vi "Timer enkoder update.vi"(7 "Akcja (Get T)":T1=enum."Get Time", 8 "error in (no error)":errorcluster, 10 "Set Time":dbl) -> (0 "error out":errorcluster, 2 "Get Time":dbl, 3 "Elapsed?":bool)   [LabVIEW 2014]
doc: "Use this template to build a VI to use as a subVI."
uses:
  Kontrolki/FVGs/FGV Timer akcje.ctl
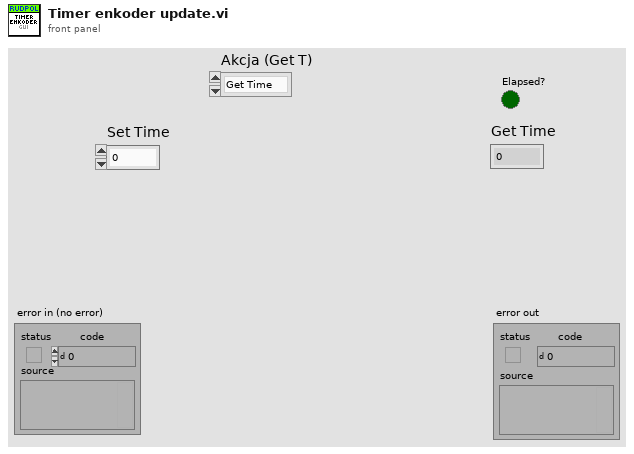
[diagram p1: front panel]
types:
  T1 = typedef "FGV Timer akcje.ctl" = enum16{"Reset", "Get Time"}
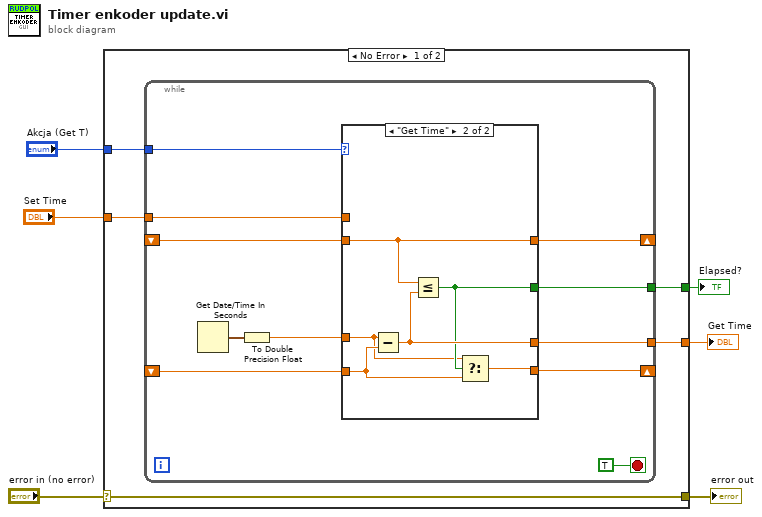
[diagram p0: block diagram]
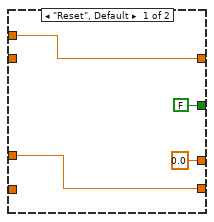
[diagram p2: hidden frame]
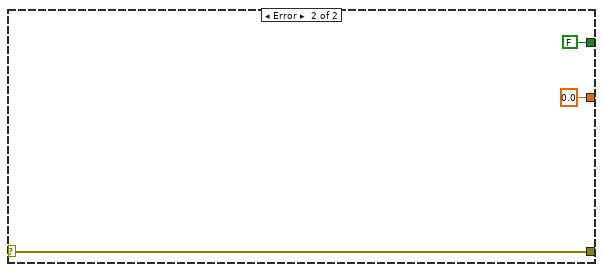
[diagram p3: hidden frame]
diagram:
  n1 = case shown="No Error" "error in (no error)" {
    selector: "error in (no error)" -> [w11 w35]
    tunnel: [w11 w35] -> w5
    tunnel: "Akcja (Get T)" -> [w10 _]
    tunnel: "Set Time" -> [w9 _]
    tunnel: [w8 0.0] -> w2
    tunnel: [w7 FALSE] -> w1
    frame No Error {
      n2 = while {
        tunnel: w10 -> [w22]
        tunnel: w9 -> [w19]
        shift-right: [w20] -> _
        shift-left: _ -> [w18]
        shift-right: [w15] -> _
        shift-left: _ -> [w14]
        tunnel: [w13] -> w8
        tunnel: [w12] -> w7
        stop <- TRUE stop-if-true
        n3 = Get Date/Time In Seconds() -> (seconds since 1Jan1904=w17:timestamp)
        n4 = To Double Precision Float(number=w17) -> (double precision float=w16:dbl)
        n5 = case shown="\"Get Time\"" w22 {
          tunnel: [w26 w32] -> w20
          tunnel: w19 -> [w26 _]
          tunnel: w18 -> [_ w32]
          tunnel: w16 -> [w25 w27]
          tunnel: [w25 w28] -> w15
          tunnel: w14 -> [_ w29]
          tunnel: [0.0 w31] -> w13
          tunnel: [FALSE w30] -> w12
          frame "Reset", Default {
          }
          frame "Get Time" {
            n6 = Subtract(x=w27, y=w29) -> (x-y=w31:dbl)
            n7 = Less Or Equal?(x=w32, y=w31) -> (x <= y?=w30:bool)
            n8 = Select(t=w27, s=w30, f=w29) -> (s? t:f=w28:dbl)
          }
        }
      }
    }
    frame Error {
    }
  }
  "error out" <- w5
  "Get Time" <- w2
  "Elapsed?" <- w1
